vi "GetVessels.vi"(8 "error in (no error)":errorcluster, 9 "Position":dbl[](array[numeric]), 10 "condition":string, 11 "Database in":refnum<class "Database.lvclass">) -> (0 "error out":errorcluster, 2 "Vessel Cluster":T1, 3 "Database out":refnum<class "Database.lvclass">)   [LabVIEW 2012, in "Database.lvclass"]
uses:
  Database.lvclass
  Database.lvclass/Database.ctl
  <vilib>/addons/database/_DB Variant To Data/Database Variant To Data.xnode
  <vilib>/addons/database/NI_Database_API.lvlib
panel:
  out "looking for file:":path
  in  "Default Pos":dbl[](array[numeric])
  in  "Cluster":T1
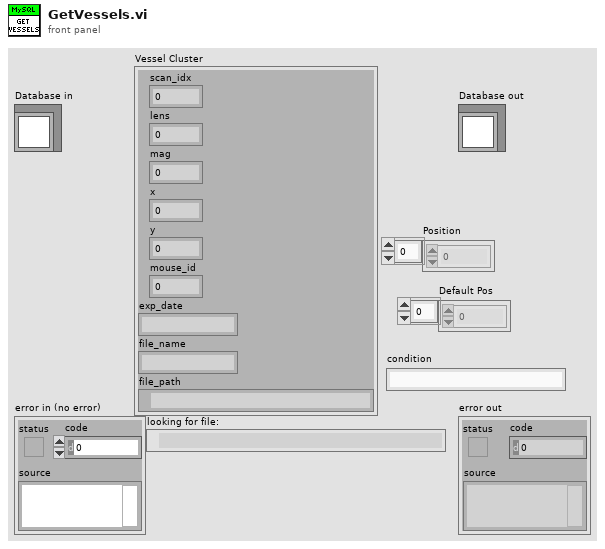
[diagram p1: front panel]
types:
  T1 = cluster{"scan_idx":i32, "lens":i32, "mag":dbl, "x":dbl, "y":dbl, "mouse_id":i32, "exp_date":string, "file_name":string, "file_path":path}
  T2 = typedef "NI_Database_API.lvlib/Conn ObjectReference.ctl" = refnum<k1>
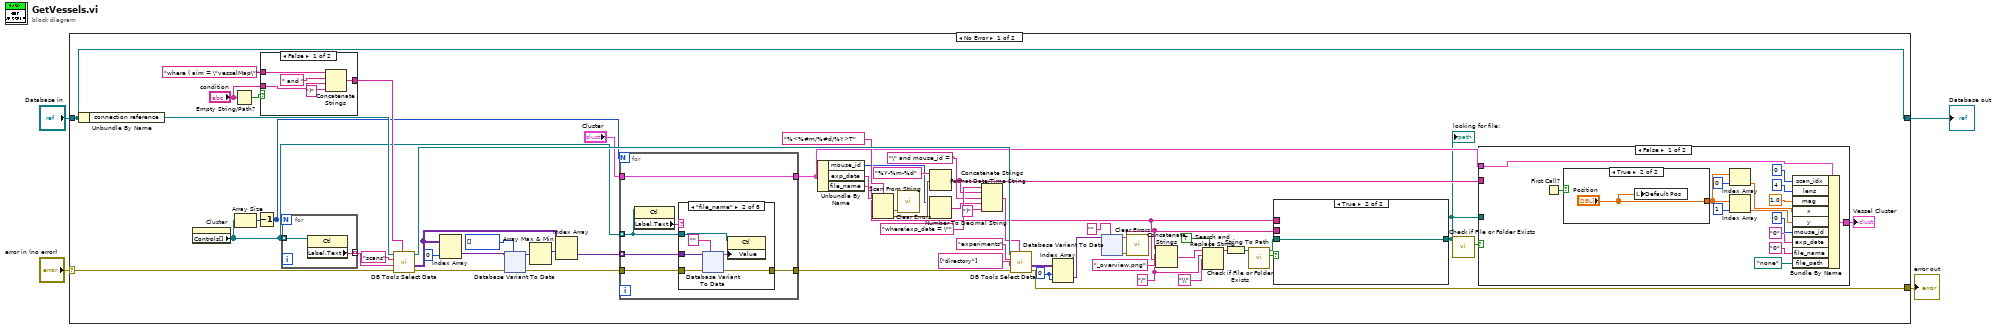
[diagram p0: block diagram]
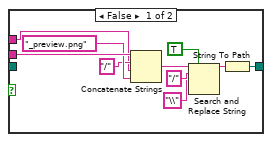
[diagram p2: hidden frame]
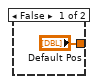
[diagram p3: hidden frame]
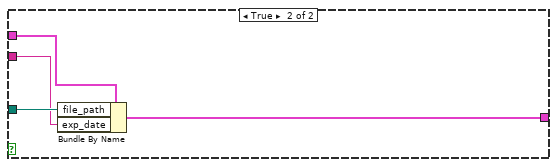
[diagram p4: hidden frame]
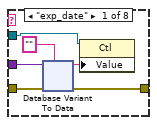
[diagram p5: hidden frame]
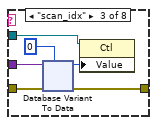
[diagram p6: hidden frame]
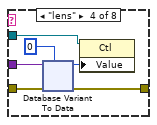
[diagram p7: hidden frame]
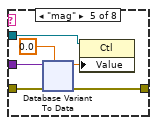
[diagram p8: hidden frame]
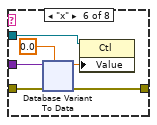
[diagram p9: hidden frame]
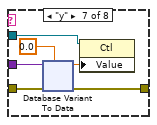
[diagram p10: hidden frame]
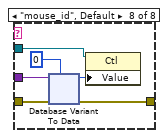
[diagram p11: hidden frame]
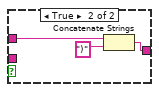
[diagram p12: hidden frame]
diagram:
  n1 = case shown="No Error" "error in (no error)" {
    selector: "error in (no error)" -> [w51 w487]
    tunnel: [w17 w487] -> w3
    tunnel: [w62 w486] -> w1
    tunnel: "Database in" -> [w62 w486]
    frame No Error {
      w7 = "/" ("search string")
      w34 = 0 ("index (row)")
      n2 = Unbundle By Name(w62) -> ("connection reference"=w61:T2)
      n3 = property on="Cluster" class="Clust (strict)"() -> ("Controls[]"=w49:refnum<vi>[])  [unwired: 2 in, 2 out]
      n4 = Empty String/Path?(string/path="condition") -> (empty?=w59:bool)
      n5 = Array Size(array=w49) -> (size(s)=w54:i32)
      n6 = Decrement(x=w54) -> (x-1=w48:i32)
      n7 = case shown="False" w59 {
        tunnel: "where ( aim = \"vesselMap\"" ("condition") -> [w482 w484]
        tunnel: [w478 w483] -> w57
        tunnel: "condition" -> [w480 _]
        frame False {
          n8 = Concatenate Strings(w482, " and ", w480, ")" ("string")) -> (w478:string)
        }
        frame True {
          n9 = Concatenate Strings(w484, ")" ("string")) -> (w483:string)
        }
      }
      n10 = for {
        N: w48 -> [_]
        tunnel: w49 -> [w477] mode=indexing
        tunnel: [w476] -> w52 mode=indexing
        n11 = property class="Ctl"(reference=w477) -> ("Label.Text"=w476:string)  [unwired: 1 in, 2 out]
      }
      n12 = call <vilib>:"DB Tools Select Data.vi"("condition"=w57, "error in (no error)"=w51, "columns"=w52, "table"="scans", "connection reference"=w61) -> ("error out"=w47:errorcluster, "data"=w53:variant[][], "connection reference out"=w55:T2)  [unwired: 1 in]
      n13 = Index Array(array=w53, index (col)=0 ("disabled index (col)")) -> (element=w45:variant[])  [unwired: 1 in]
      n14 = xnode "Database Variant To Data"("database variant"=w45, "error in"=w47, "type"=i32[] []) -> ("data"=w43:i32[], "error out"=w22:errorcluster)
      n15 = Array Max & Min(array=w43) -> (max index (indices)=w28:i32)  [unwired: 3 out]
      n16 = Index Array(array=w53, index (row)=w28) -> (element=w27:variant[])  [unwired: 1 in]
      n17 = for {
        N: w48 -> [_]
        tunnel: w49 -> [w98] mode=indexing
        tunnel: w27 -> [w101] mode=indexing
        tunnel: "Cluster" -> [w100]
        tunnel: [w100] -> w24
        tunnel: w22 -> [w97]
        tunnel: [w96] -> w21
        n18 = property class="Ctl"(reference=w98) -> ("Label.Text"=w99:string)  [unwired: 1 in, 2 out]
        n19 = case shown="\"file_name\"" w99 {
          tunnel: w101 -> [w107 w144 w181 w218 w256 w294 w333 w371]
          tunnel: w98 -> [w106 w142 w182 w219 w257 w295 w332 w370]
          tunnel: w97 -> [w103 w141 w179 w217 w255 w293 w331 w369]
          tunnel: [w102 w140 w178 w216 w254 w292 w330 w368] -> w96
          frame "exp_date" {
            n20 = xnode "Database Variant To Data"("database variant"=w107, "error in"=w103, "type"="") -> ("data"=w104:string, "error out"=w102:errorcluster)
            n21 = property class="Ctl"(reference=w106, "Value"=w104) -> ()  [unwired: 1 in, 2 out]
          }
          frame "file_name" {
            n22 = xnode "Database Variant To Data"("database variant"=w144, "error in"=w141, "type"="") -> ("data"=w145:string, "error out"=w140:errorcluster)
            n23 = property class="Ctl"(reference=w142, "Value"=w145) -> ()  [unwired: 1 in, 2 out]
          }
          frame "scan_idx" {
            n24 = xnode "Database Variant To Data"("database variant"=w181, "error in"=w179, "type"=0) -> ("data"=w183:i32, "error out"=w178:errorcluster)
            n25 = property class="Ctl"(reference=w182, "Value"=w183) -> ()  [unwired: 1 in, 2 out]
          }
          frame "lens" {
            n26 = xnode "Database Variant To Data"("database variant"=w218, "error in"=w217, "type"=0) -> ("data"=w221:i32, "error out"=w216:errorcluster)
            n27 = property class="Ctl"(reference=w219, "Value"=w221) -> ()  [unwired: 1 in, 2 out]
          }
          frame "mag" {
            n28 = xnode "Database Variant To Data"("database variant"=w256, "error in"=w255, "type"=0.0) -> ("data"=w259:dbl, "error out"=w254:errorcluster)
            n29 = property class="Ctl"(reference=w257, "Value"=w259) -> ()  [unwired: 1 in, 2 out]
          }
          frame "x" {
            n30 = xnode "Database Variant To Data"("database variant"=w294, "error in"=w293, "type"=0.0) -> ("data"=w297:dbl, "error out"=w292:errorcluster)
            n31 = property class="Ctl"(reference=w295, "Value"=w297) -> ()  [unwired: 1 in, 2 out]
          }
          frame "y" {
            n32 = xnode "Database Variant To Data"("database variant"=w333, "error in"=w331, "type"=0.0) -> ("data"=w335:dbl, "error out"=w330:errorcluster)
            n33 = property class="Ctl"(reference=w332, "Value"=w335) -> ()  [unwired: 1 in, 2 out]
          }
          frame "mouse_id", Default {
            n34 = xnode "Database Variant To Data"("database variant"=w371, "error in"=w369, "type"=i16 0) -> ("data"=w373:i16, "error out"=w368:errorcluster)
            n35 = property class="Ctl"(reference=w370, "Value"=w373) -> ()  [unwired: 1 in, 2 out]
          }
        }
      }
      n36 = Unbundle By Name(w24) -> ("mouse_id"=w26:i32, "exp_date"=w25:string, "file_name"=w6:string)
      n37 = Scan From String(format string="%<%#m/%#d/%Y>T" ("input string"), input string=w25) -> (error out=w18:errorcluster, output 1=w30:timestamp)  [unwired: 2 in, 3 out]
      n38 = call <vilib>:"Clear Errors.vi"("error in (no error)"=w18) -> ()  [unwired: 6 in, 1 out]
      n39 = Format Date/Time String(time format string (%c)="%Y-%m-%d", seconds (now)=w30) -> (date/time string=w23:string)  [unwired: 1 in]
      n40 = Number To Decimal String(number=w26) -> (decimal integer string=w37:string)  [unwired: 1 in]
      n41 = Concatenate Strings("where(exp_date = \"" ("string"), w23, "\" and mouse_id = " ("string"), w37, ")" ("string")) -> (w36:string)
      n42 = call <vilib>:"DB Tools Select Data.vi"("condition"=w36, "error in (no error)"=w21, "columns"=string[] ["directory"], "table"="experiments", "connection reference"=w55) -> ("error out"=w17:errorcluster, "data"=w35:variant[][])  [unwired: 1 in, 1 out]
      n43 = Index Array(array=w35, index (row)=w34, index (col)=w34) -> (element=w33:variant)
      n44 = xnode "Database Variant To Data"("database variant"=w33, "type"="") -> ("data"=w8:string, "error out"=w16:errorcluster)  [unwired: 1 in]
      n45 = call <vilib>:"Clear Errors.vi"("error in (no error)"=w16) -> ()  [unwired: 6 in, 1 out]
      n46 = Concatenate Strings(w8, w7, w6, "_overview.png" ("string")) -> (w11:string)
      n47 = Search and Replace String(replace all?=TRUE ("replace all? (F)"), input string=w11, search string=w7, replace string="\\" ("replace string (\"\")")) -> (result string=w13:string)  [unwired: 4 in, 3 out]
      n48 = String To Path(string=w13) -> (path=w15:path)
      n49 = call <vilib>:"Check if File or Folder Exists.vi"("path"=w15) -> ("file or folder exists?"=w9:bool, "dup path"=w5:path)  [unwired: 8 in, 1 out]
      n50 = case shown="True" w9 {
        tunnel: w8 -> [w73 _]
        tunnel: w6 -> [w65 _]
        tunnel: [w64 w74] -> w20
        tunnel: w5 -> [_ w74]
        frame False {
          n51 = Concatenate Strings(w73, "/" ("string"), w65, "_preview.png" ("string")) -> (w70:string)
          n52 = Search and Replace String(replace all?=TRUE ("replace all? (F)"), input string=w70, search string="/", replace string="\\" ("replace string (\"\")")) -> (result string=w67:string)  [unwired: 4 in, 3 out]
          n53 = String To Path(string=w67) -> (path=w64:path)
        }
        frame True {
        }
      }
      "looking for file:" <- w20
      n54 = call <vilib>:"Check if File or Folder Exists.vi"("path"=w20) -> ("file or folder exists?"=w19:bool)  [unwired: 8 in, 2 out]
      n55 = case shown="False" w19 {
        tunnel: [w83 w95] -> w46
        tunnel: w20 -> [_ w94]
        tunnel: w24 -> [w82 w93]
        tunnel: w23 -> [_ w92]
        frame False {
          n56 = First Call?() -> (First Call?: T/F=w75:bool)
          n57 = case shown="True" w75 {
            tunnel: ["Default Pos" "Position"] -> w80
            frame False {
            }
            frame True {
              n58 = local write "Default Pos"("Position") -> ()
            }
          }
          n59 = Index Array(array=w80, index=0) -> (element=w77:dbl)
          n60 = Index Array(array=w80, index=1) -> (element=w76:dbl)
          n61 = Bundle By Name(cluster=w82, "scan_idx"=0, "lens"=4, "mag"=1.0, "x"=w77, "y"=w76, "mouse_id"=0, "exp_date"="0", "file_name"="0", "file_path"=path "none") -> (w83:T1)
        }
        frame True {
          n62 = Bundle By Name(cluster=w93, "file_path"=w94, "exp_date"=w92) -> (w95:T1)
        }
      }
      "Vessel Cluster" <- w46
    }
    frame Error {
    }
  }
  "error out" <- w3
  "Database out" <- w1
